vi "DisplayArrayOfPictures.vi"(3 "stop":bool, 4 "Array Of Pictures":picture[](array[picture])) -> (0 "Picture 3":picture, 1 "Picture 2":picture, 2 "Picture":picture)   [LabVIEW 2013]
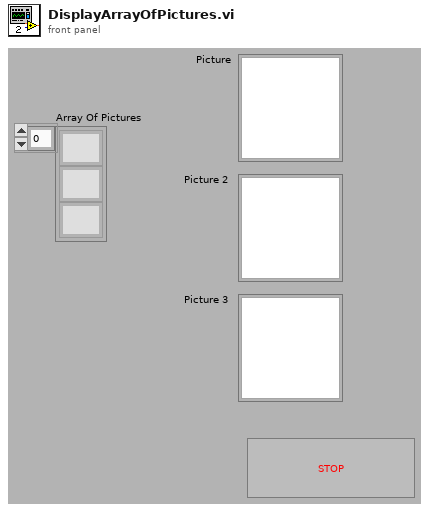
[diagram p1: front panel]
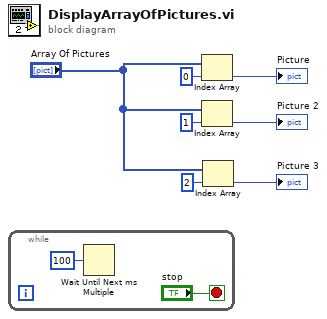
[diagram p0: block diagram]
diagram:
  n1 = while {
    stop <- "stop" stop-if-true
    n2 = Wait Until Next ms Multiple(millisecond multiple=u32 100) -> ()  [unwired: 1 out]
  }
  n3 = Index Array(array="Array Of Pictures", index=0) -> (element=→"Picture":picture)
  n4 = Index Array(array="Array Of Pictures", index=1) -> (element=→"Picture 2":picture)
  n5 = Index Array(array="Array Of Pictures", index=2) -> (element=→"Picture 3":picture)
